vi "picoquant_receive_data_for_processing.vi"(8 "error in (no error)":errorcluster, 11 "picoquant_generic in":refnum<class "picoquant_generic.lvclass">) -> (0 "error out":errorcluster, 1 "timed out?":bool, 2 "data_out":T1, 3 "picoquant_generic out":refnum<class "picoquant_generic.lvclass">)   [LabVIEW 2015, in "picoquant_generic.lvclass"]
uses:
  picoquant_generic.lvclass
  picoquant_data_tdef.ctl
  picoquant_generic.lvclass/picoquant_generic.ctl
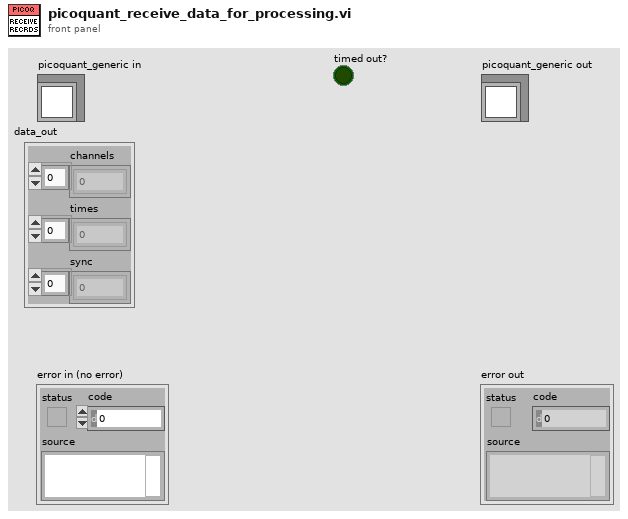
[diagram p1: front panel]
types:
  T1 = typedef "picoquant_data_tdef.ctl" = cluster{"channels":u8[], "times":u64[], "sync":u64[]}
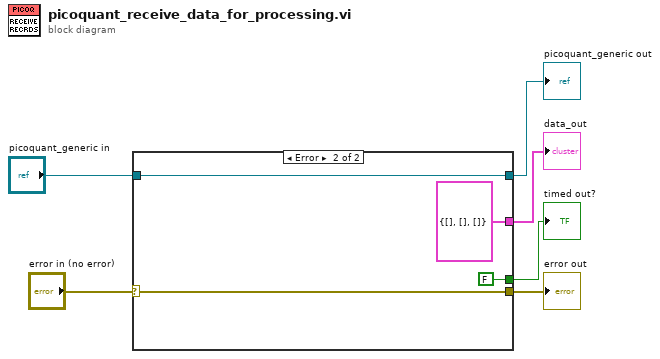
[diagram p0: block diagram]
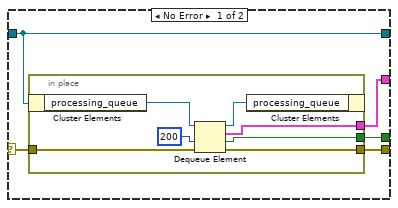
[diagram p2: hidden frame]
diagram:
  n1 = case shown="Error" "error in (no error)" {
    selector: "error in (no error)" -> [w10 w22]
    tunnel: [w7 w22] -> w5
    tunnel: [w11 w21] -> w3
    tunnel: "picoquant_generic in" -> [w11 w21]
    tunnel: [w9 T1 {"channels"=[], "times"=[], "sync"=[]} ("process_data")] -> w2
    tunnel: [w8 FALSE ("timed out?")] -> w1
    frame No Error {
      n2 = in-place {
        in-place-border: w10 -> [w16]
        in-place-border: [w14] -> w9
        in-place-border: [w13] -> w8
        in-place-border: [w12] -> w7
        n3 = in-place-cluster #1(w11) -> ("processing_queue"=w18:refnum<queue>)
        n4 = Dequeue Element(queue=w18, timeout in ms (-1)=200, error in (no error)=w16) -> (queue out=w15:refnum<queue>, element=w14:T1, timed out?=w13:bool, error out=w12:errorcluster)
        n5 = in-place-cluster #1("processing_queue"=w15) -> ()  [unwired: 1 out]
      }
    }
    frame Error {
    }
  }
  "error out" <- w5
  "picoquant_generic out" <- w3
  "data_out" <- w2
  "timed out?" <- w1
